vi "BU-Process-KLaws.vi"(11 "Original Set of equations":string[][](table)) -> (2 "Output Equations w param":string[][](table), 3 "Output Equations":string[][](table))   [LabVIEW 2014]
panel:
  out "UCF Param":string[][](table)
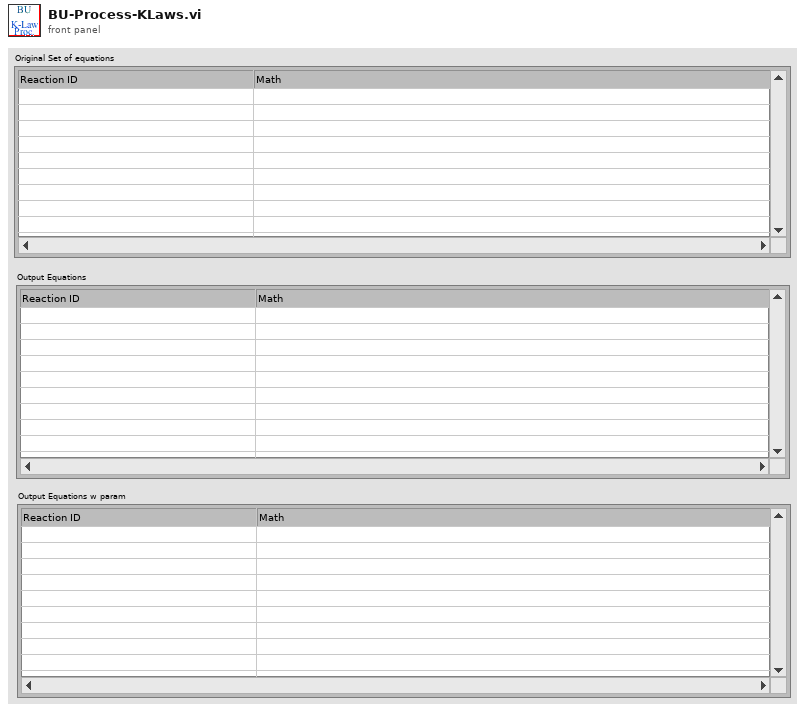
[diagram p1: front panel]
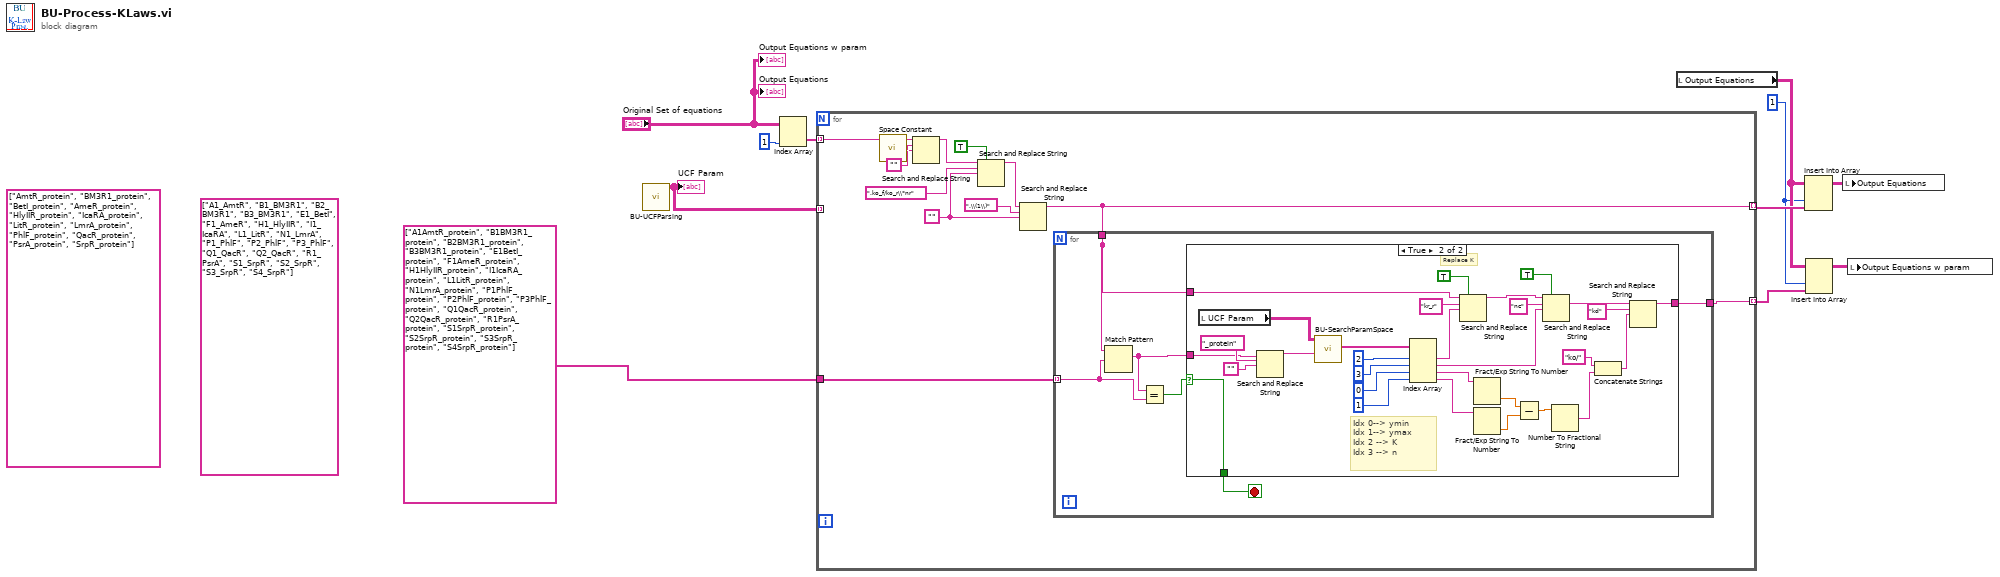
[diagram p0: block diagram]
diagram:
  (unwired) string[] ["A1_AmtR", "B1_BM3R1", "B2_BM3R1", "B3_BM3R1", "E1_BetI", "F1_AmeR", "H1_HlyIIR", "I1_IcaRA", "L1_LitR", "N1_LmrA", "P1_PhlF", "P2_PhlF", "P3_PhlF", "Q1_QacR", "Q2_QacR", "R1_PsrA", "S1_SrpR", "S2_SrpR", "S3_SrpR", "S4_SrpR"] ("string array")
  (unwired) string[] ["AmtR_protein", "BM3R1_protein", "BetI_protein", "AmeR_protein", "HlyIIR_protein", "IcaRA_protein", "LitR_protein", "LmrA_protein", "PhlF_protein", "QacR_protein", "PsrA_protein", "SrpR_protein"] ("string array")
  w6 = 1 ("disabled index (col)")
  n1 = call "BU-UCFParsing.vi"() -> ("Gate values"=w2:string[][])  [unwired: 11 in]
  "UCF Param" <- w2
  n2 = Index Array(array="Original Set of equations", index (col)=1 ("disabled index (col)")) -> (element=w10:string[])  [unwired: 1 in]
  n3 = for {
    tunnel: w10 -> [w23] mode=indexing
    tunnel: [w13] -> w8 mode=indexing
    tunnel: string[] ["A1AmtR_protein", "B1BM3R1_protein", "B2BM3R1_protein", "B3BM3R1_protein", "E1BetI_protein", "F1AmeR_protein", "H1HlyIIR_protein", "I1IcaRA_protein", "L1LitR_protein", "N1LmrA_protein", "P1PhlF_protein", "P2PhlF_protein", "P3PhlF_protein", "Q1QacR_protein", "Q2QacR_protein", "R1PsrA_protein", "S1SrpR_protein", "S2SrpR_protein", "S3SrpR_protein", "S4SrpR_protein"] ("string array") -> [w14]
    tunnel: [w12] -> w5 mode=indexing
    tunnel: w2 -> [_] mode=indexing
    w15 = ""
    n4 = call <vilib>:"Space Constant.vi"() -> ("String"=w22:string)
    n5 = Search and Replace String(input string=w23, search string=w22, replace string="") -> (result string=w19:string)  [unwired: 5 in, 3 out]
    n6 = Search and Replace String(replace all?=TRUE ("replace all? (F)"), input string=w19, search string=".ko_f/ko_r\\*nr" ("regular expression"), replace string=w15) -> (result string=w17:string)  [unwired: 4 in, 3 out]
    n7 = Search and Replace String(input string=w17, search string=".\\(1\\)" ("regular expression"), replace string=w15) -> (result string=w13:string)  [unwired: 5 in, 3 out]
    n8 = for {
      tunnel: w14 -> [w28] mode=indexing
      tunnel: w13 -> [w27]
      tunnel: [w26] -> w12
      stop <- w24 stop-if-true
      n9 = Match Pattern(string=w27, regular expression=w28) -> (match substring=w29:string)  [unwired: 1 in, 3 out]
      n10 = Equal?(x=w29, y=w28) -> (x = y?=w25:bool)
      n11 = case shown="True" w25 {
        selector: w25 -> [w31 w38]
        tunnel: w29 -> [_ w59]
        tunnel: w27 -> [w30 w53]
        tunnel: [w30 w36] -> w26
        tunnel: [w31 w38] -> w24
        frame False {
        }
        frame True {
          # "Replace K"
          # "Idx 0--> ymin\nIdx 1--> ymax\nIdx 2 --> K\nIdx 3 --> n"
          n12 = local read "UCF Param"() -> (w58:string[][])
          n13 = Search and Replace String(input string=w59, search string="_protein", replace string="") -> (result string=w57:string)  [unwired: 5 in, 3 out]
          n14 = call "BU-SearchParamSpace.vi"("Input String"=w57, "UCF Param"=w58) -> ("Req Param"=w56:string[])  [unwired: 9 in]
          n15 = Index Array(array=w56, index #1=2 ("index"), index #2=3 ("index"), index #3=0 ("index"), index #4=1 ("index")) -> (element #1=w51:string, element #2=w48:string, element #3=w42:string, element #4=w41:string)
          n16 = Search and Replace String(replace all?=TRUE ("replace all? (F)"), input string=w53, search string="kr_r", replace string=w51) -> (result string=w49:string)  [unwired: 4 in, 3 out]
          n17 = Fract/Exp String To Number(string=w42) -> (number=w40:dbl)  [unwired: 3 in, 1 out]
          n18 = Fract/Exp String To Number(string=w41) -> (number=w39:dbl)  [unwired: 3 in, 1 out]
          n19 = Subtract(x=w40, y=w39) -> (x-y=w35:dbl)
          n20 = Search and Replace String(replace all?=TRUE ("replace all? (F)"), input string=w49, search string="nc", replace string=w48) -> (result string=w45:string)  [unwired: 4 in, 3 out]
          n21 = Number To Fractional String(number=w35) -> (F-format string=w33:string)  [unwired: 3 in]
          n22 = Concatenate Strings("ko/" ("search string"), w33) -> (w32:string)
          n23 = Search and Replace String(input string=w45, search string="kd", replace string=w32) -> (result string=w36:string)  [unwired: 5 in, 3 out]
        }
      }
    }
  }
  n24 = local read "Output Equations"() -> (w7:string[][])
  n25 = Insert Into Array(array=w7, index (col)=w6, new element=w8) -> (w9:string[][])  [unwired: 1 in]
  n26 = Insert Into Array(array=w7, index (col)=w6, new element=w5) -> (w3:string[][])  [unwired: 1 in]
  n27 = local write "Output Equations"(w9) -> ()
  n28 = local write "Output Equations w param"(w3) -> ()
  "Output Equations" <- "Original Set of equations"
  "Output Equations w param" <- "Original Set of equations"
